vi "예제1.vi"() -> ()   [LabVIEW 2020]
panel:
  out "수신 차트":dbl(graph)
  out "송신 차트":dbl(graph)
  in  "정지":bool
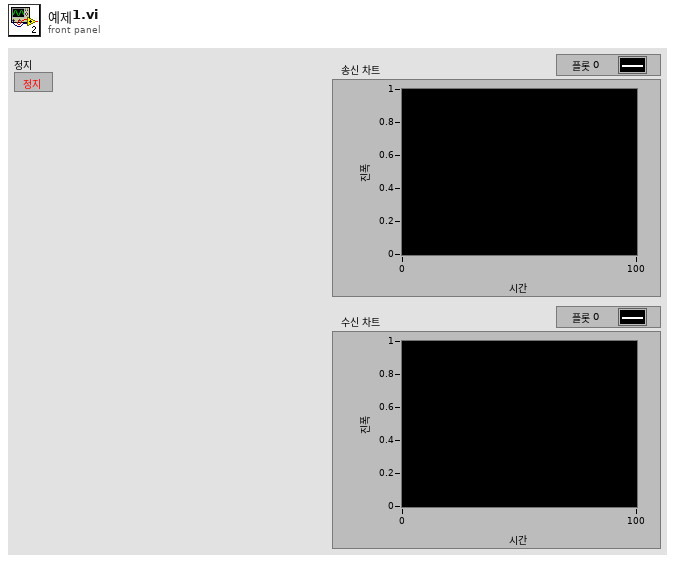
[diagram p1: front panel]
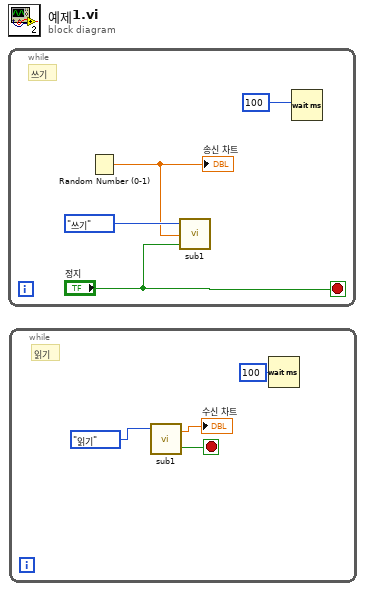
[diagram p0: block diagram]
diagram:
  n1 = while {
    stop <- "정지" stop-if-true
    # "쓰기"
    n2 = Random Number (0-1)() -> (number: 0 to 1=w2:dbl)
    "송신 차트" <- w2
    n3 = call "sub1.vi"("정지 In"="정지", "데이터 In"=w2, "FGV 상태"=enum16{"쓰기", "읽기"}."쓰기") -> ()  [unwired: 2 out]
    n4 = Wait (ms)(milliseconds to wait=u32 100 ("ms 타이머 값")) -> ()  [unwired: 1 out]
  }
  n5 = while {
    stop <- w8 stop-if-true
    # "읽기"
    n6 = call "sub1.vi"("FGV 상태"=enum16{"쓰기", "읽기"}."읽기") -> ("정지 Out"=w8:bool, "데이터 Out"=→"수신 차트":dbl)  [unwired: 2 in]
    n7 = Wait (ms)(milliseconds to wait=u32 100 ("ms 타이머 값")) -> ()  [unwired: 1 out]
  }
